vi "Read RSS Feed.vi"() -> ()   [LabVIEW 2011]
panel:
  in  "URL":string="http://forums.lavag.org/rss-8.html"
  out "rss":T1
  out "raw rss data":string
  # "Run this VI to download the RSS file and load it into the indicators below"
  # "1) download from Internet"
  # "2) parse raw rss data into LabVIEW data"
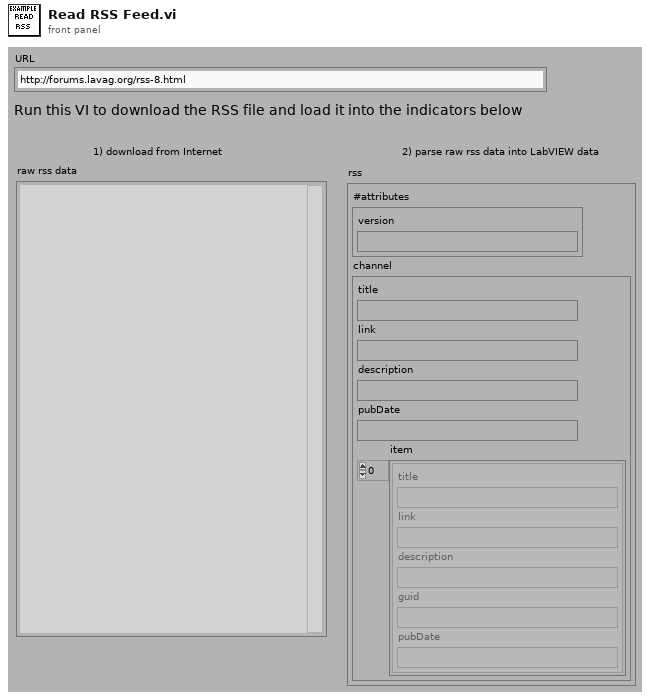
[diagram p1: front panel]
types:
  T1 = cluster{"#attributes":cluster{"version":string}, "channel":cluster{"title":string, "link":string, "description":string, "pubDate":string, "item":cluster{"title":string, "link":string, "description":string, "guid":string, "pubDate":string}[]}}
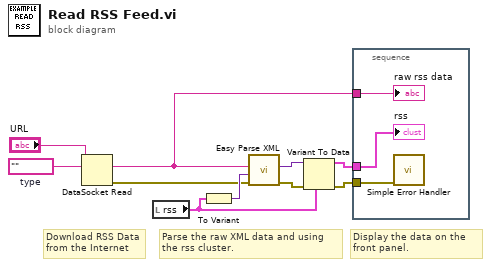
[diagram p0: block diagram]
diagram:
  w7 = ""  # type
  # "Display the data on the front panel."
  # "Parse the raw XML data and using the rss cluster."
  # "Download RSS Data from the Internet"
  n1 = DataSocket Read(10:w7, 11:"URL") -> (0:w2:errorcluster, 2:w1:string)  [unwired: 3 in, 5 out]
  n2 = local read "rss"() -> (w10:T1)
  n3 = To Variant(anything=w10) -> (Variant=w5:variant)
  n4 = call "Easy Parse XML.vi"("error in (no error)"=w2, "LabVIEW Data (Type)"=w5, "XML String"=w1) -> ("error out"=w3:errorcluster, "LabVIEW Data"=w4:variant)  [unwired: 7 in]
  n5 = Variant To Data(error in=w3, type=w10, Variant=w4) -> (data=w9:T1, error out=w8:errorcluster)
  n6 = stacked-sequence {
    tunnel: w9 -> [w13]
    tunnel: w8 -> [w12]
    tunnel: w1 -> [w11]
    frame #0 {
      n7 = call <vilib>:"Simple Error Handler.vi"("error in (no error)"=w12) -> ()  [unwired: 4 in, 5 out]
      "raw rss data" <- w11
      "rss" <- w13
    }
  }
